vi "Configure Archiving Dialog.vi"(8 "error in (no error)":errorcluster, 11 "System Configuration In":T1={"Name"="Chamber1", "Description"="", "Logging Computer Name"="", "Logging Database Name"="", "Logging Database Path"=path "", "Archive Computer Name"="", "Archive Database Name"="", "Archive Database Path"=path "", "Lifespan (days)"=0, "Archive Enabled"=FALSE, "Archive Interval (hours)"=0, "Subsystems"=[]}) -> (0 "error out":errorcluster, 2 "Changed?":bool, 3 "System Configuration Out":T1={"Name"="Chamber1", "Description"="", "Logging Computer Name"="", "Logging Database Name"="", "Logging Database Path"=path "", "Archive Computer Name"="", "Archive Database Name"="", "Archive Database Path"=path "", "Lifespan (days)"=0, "Archive Enabled"=FALSE, "Archive Interval (hours)"=0, "Subsystems"=[]})   [LabVIEW 2024]
doc: "This VI is a user interface VI and is used to configures data archiving."
uses:
  Controls/Server/System Configuration.ctl
  Controls/Server/Subsystem Configuration.ctl
panel:
  in  "Archive Computer Name":string
  in  "Archive Enabled":bool
  in  "Archive Database Path":path
  in  "Archive Database Name":string
  in  "Archive Interval (hours)":u32=24 min=1 max=10000 step=1
  in  "Cancel":bool
  in  "OK":bool
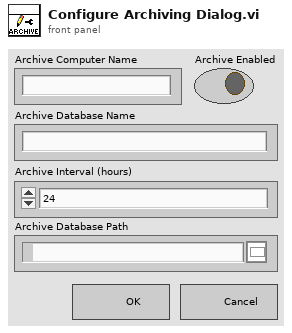
[diagram p1: front panel]
types:
  T1 = typedef "System Configuration.ctl" = cluster{"Name":string, "Description":string, "Logging Computer Name":string, "Logging Database Name":string, "Logging Database Path":path, "Archive Computer Name":string, "Archive Database Name":string, "Archive Database Path":path, "Lifespan (days)":u32, "Archive Enabled":bool, "Archive Interval (hours)":u32, "Subsystems":T2[]}
  T2 = typedef "Subsystem Configuration.ctl" = cluster{"Name":string, "Root URL":refnum<k21>}
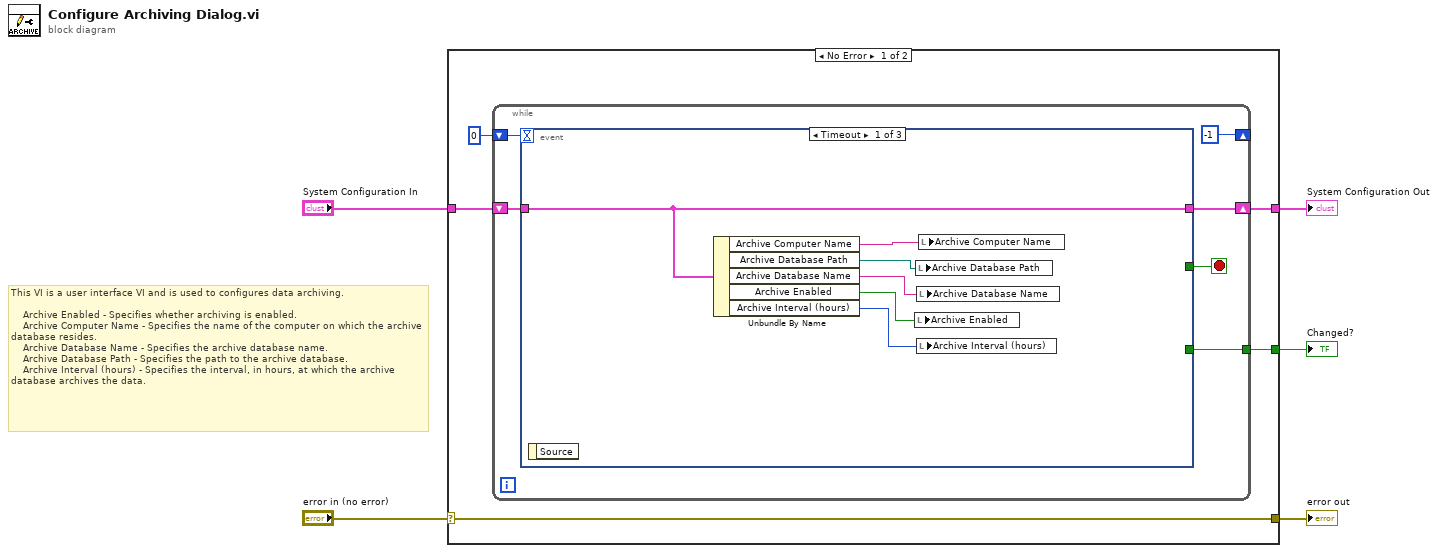
[diagram p0: block diagram]
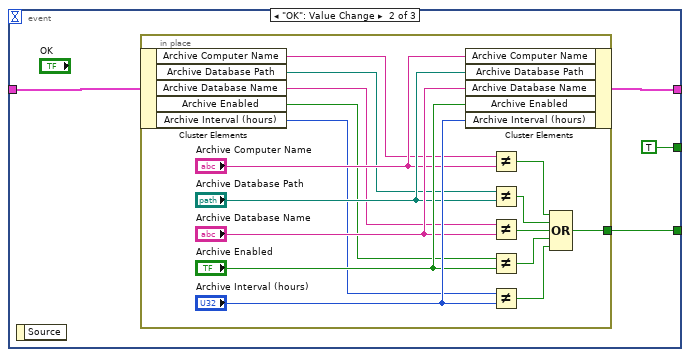
[diagram p2: hidden frame]
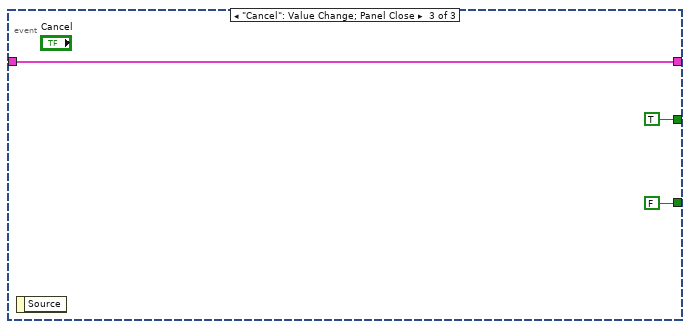
[diagram p3: hidden frame]
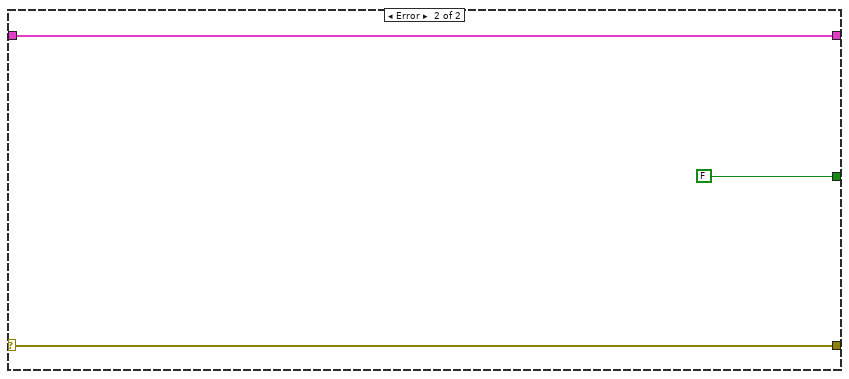
[diagram p4: hidden frame]
diagram:
  # "This VI is a user interface VI and is used to configures data archiving.\n\n    Archive Enabled - Specifies whether archiving is enabled.\n    Archive Computer Name - Specifies the name of the computer on which the archive database resides. \n    Archive Database Name - Specifies the archive database name. \n    Archive Database Path - Specifies the path to the archive database. \n    Archive Interval (hours) - Specifies the interval, in hours, at which the archive database archives the data."
  n1 = case shown="No Error" "error in (no error)" {
    selector: "error in (no error)" -> [w10 w48]
    tunnel: [w10 w48] -> w4
    tunnel: [w8 FALSE ("UI Refresh Needed?")] -> w1
    tunnel: "System Configuration In" -> [w6 w47]
    tunnel: [w9 w47] -> w2
    frame No Error {
      n2 = while {
        tunnel: [w16] -> w8
        shift-right: [w14] -> w9
        shift-left: w6 -> [w15]
        shift-right: [-1] -> _
        shift-left: 0 -> [w12]
        stop <- w13 stop-if-true
        n3 = event shown="[0] Timeout" {
          selector: _ -> [_ _ _]
          dyn-events: _ -> [_ _ _]
          timeout: w12 -> [_ _ _]
          tunnel: [_ w23 FALSE ("UI Refresh Needed?")] -> w16
          tunnel: w15 -> [w17 w25 w43]
          tunnel: [w17 w24 w43] -> w14
          tunnel: [_ TRUE TRUE] -> w13
          event Timeout {
            n4 = event-data() -> ()  [unwired: 1 in, 1 out]
            n5 = Unbundle By Name(w17) -> ("Archive Computer Name"=w22:string, "Archive Database Path"=w18:path, "Archive Database Name"=w21:string, "Archive Enabled"=w19:bool, "Archive Interval (hours)"=w20:u32)
            n6 = local write "Archive Enabled"(w19) -> ()
            n7 = local write "Archive Database Path"(w18) -> ()
            n8 = local write "Archive Database Name"(w21) -> ()
            n9 = local write "Archive Interval (hours)"(w20) -> ()
            n10 = local write "Archive Computer Name"(w22) -> ()
          }
          event "OK": Value Change {
            n11 = event-data() -> ()  [unwired: 1 in, 1 out]
            n12 = in-place {
              in-place-border: [w27] -> w23
              n13 = in-place-cluster #1(w25) -> ("Archive Computer Name"=w37:string, "Archive Database Path"=w36:path, "Archive Database Name"=w35:string, "Archive Enabled"=w34:bool, "Archive Interval (hours)"=w33:u32)
              n14 = in-place-cluster #1("Archive Computer Name"="Archive Computer Name", "Archive Database Path"="Archive Database Path", "Archive Database Name"="Archive Database Name", "Archive Enabled"="Archive Enabled", "Archive Interval (hours)"="Archive Interval (hours)") -> (w24:T1)
              n15 = Not Equal?(x=w37, y="Archive Computer Name") -> (x != y?=w32:bool)
              n16 = Not Equal?(x=w36, y="Archive Database Path") -> (x != y?=w31:bool)
              n17 = Not Equal?(x=w35, y="Archive Database Name") -> (x != y?=w30:bool)
              n18 = Not Equal?(x=w34, y="Archive Enabled") -> (x != y?=w29:bool)
              n19 = Not Equal?(x=w33, y="Archive Interval (hours)") -> (x != y?=w28:bool)
              n20 = Compound Arithmetic op=OR(w32, w31, w30, w29, w28) -> (w27:bool)
            }
          }
          event "Cancel": Value Change; Panel Close {
            n21 = event-data() -> ()  [unwired: 1 in, 1 out]
          }
        }
      }
    }
    frame Error {
    }
  }
  "Changed?" <- w1
  "System Configuration Out" <- w2
  "error out" <- w4
